vi "ILABW_GetPath.vi"(11 "name":string) -> (3 "path":string)   [LabVIEW 2012]
panel:
  out "error":string
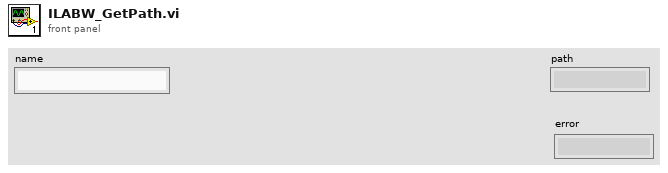
[diagram p1: front panel]
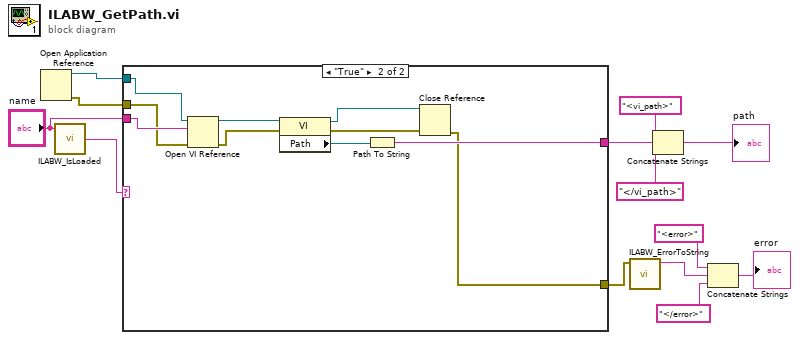
[diagram p0: block diagram]
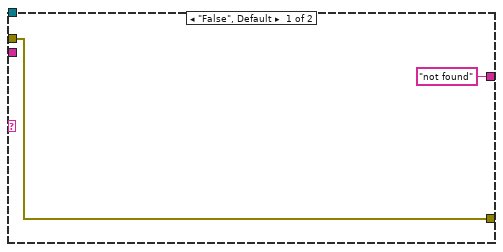
[diagram p2: hidden frame]
diagram:
  n1 = Open Application Reference() -> (0:w6:errorcluster, 3:w11:refnum<vi>)  [unwired: 4 in]
  n2 = call "ILABW_IsLoaded.vi"("name"="name") -> ("status"=w13:string)  [unwired: 2 in]
  n3 = case shown="\"True\"" w13 {
    tunnel: "name" -> [_ w25]
    tunnel: w11 -> [_ w24]
    tunnel: ["not found" w21] -> w10
    tunnel: [w14 w17] -> w1
    tunnel: w6 -> [w14 w16]
    frame "False", Default {
    }
    frame "True" {
      n4 = Open VI Reference(application reference (local)=w24, vi path=w25, error in (no error)=w16) -> (vi reference=w23:refnum<vi>, error out=w19:errorcluster)  [unwired: 3 in]
      n5 = property class="VI"(reference=w23, error in=w19) -> (reference out=w20:refnum<vi>, error out=w18:errorcluster, "Path"=w22:path)
      n6 = Path To String(path=w22) -> (string=w21:string)
      n7 = Close Reference(reference=w20, error in (no error)=w18) -> (error out=w17:errorcluster)
    }
  }
  n8 = call "ILABW_ErrorToString.vi"("errorIn"=w1) -> ("errorOut"=w2:string)  [unwired: 10 in]
  n9 = Concatenate Strings("<vi_path>" ("string"), w10, "</vi_path>" ("string")) -> (→"path":string)
  n10 = Concatenate Strings("<error>" ("string"), w2, "</error>" ("string")) -> (→"error":string)
